vi "0-Draw No-Sail Zones.vi"(4 "Font Size":i16, 5 "Image Descriptor":T2={"Upper-Left Corner Coordinates"={"UTM Zone"=0.0, "Hemisphere"=enum."North", "East"=0.0, "North"=0.0}, "Meters/Pixel"=42.294203} {"Upper-Left Corner Coordinates"."North" format="%#_10f"; "Upper-Left Corner Coordinates"."East" format="%#_8f"}, 6 "No Sail Zone Color":u32(colorbox)=16754450, 7 "No Sail Circles":T1[](array[typedef]), 8 "Image In":T4) -> (1 "Coordinate Outside Image":bool, 3 "Image Out":T4)   [LabVIEW 2011]
doc: "Overlays no-sail zones onto the map image."
uses:
  2-Think/2 Typedefs/UTM Location.ctl
  2-Think/2 Globals/2 Global.vi
  2-Think/2 Classes/Waypoint/Waypoint.lvclass
  <vilib>/vision/Image Controls.llb/IMAQ Image.ctl
  0-Image Descriptor.ctl
  2-Think/2 Typedefs/UTM Circle.ctl
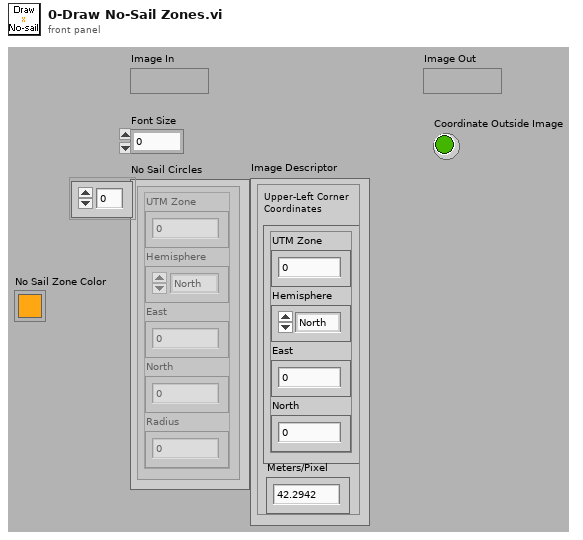
[diagram p1: front panel]
types:
  T1 = typedef "UTM Circle.ctl" = cluster{"UTM Zone":dbl, "Hemisphere":enum16{"North", "South"}, "East":dbl, "North":dbl, "Radius":dbl}
  T2 = typedef "0-Image Descriptor.ctl" = cluster{"Upper-Left Corner Coordinates":T3, "Meters/Pixel":dbl}
  T3 = typedef "UTM Location.ctl" = cluster{"UTM Zone":dbl, "Hemisphere":enum16{"North", "South"}, "East":dbl, "North":dbl}
  T4 = typedef "IMAQ Image.ctl" = refnum<image>
  T5 = cluster{"Desired Font (Application)":enum16{"User-specified Font", "Application Font", "System Font", "Dialog Font"}, "[User-specified Font]":cluster{"Font Name":string, "Size":i16, "Strikeout?":bool, "Italic?":bool, "Underline?":bool, "Outline?":bool, "Shadow?":bool, "Bold?":bool, "Rotation Angle":dbl}, "Horizontal Alignment":i16, "Vertical Alignment":i16}
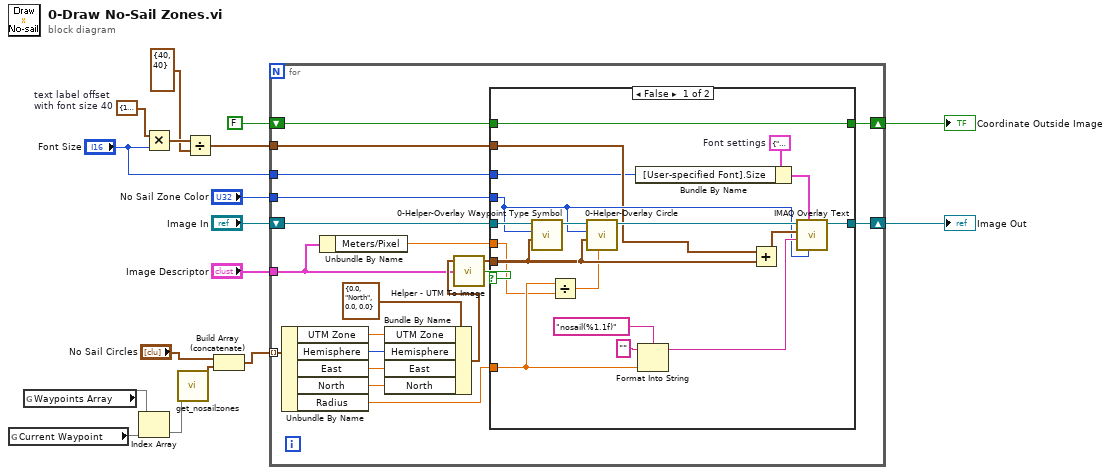
[diagram p0: block diagram]
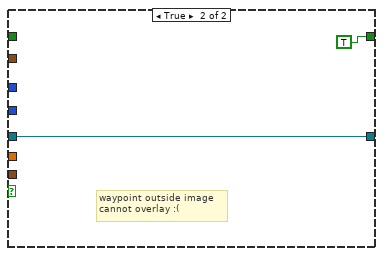
[diagram p2: hidden frame]
diagram:
  w11 = cluster{"X":i32, "Y":i32} {"X"=10, "Y"=21}  # text label offset with font size 40
  n1 = global read "2 Global.vi" "Current Waypoint"() -> (w1)
  n2 = global read "2 Global.vi" "Waypoints Array"() -> (w2)
  n3 = Index Array(array=w2, index=w1) -> (element=w3)
  n4 = Multiply(x=w11, y="Font Size") -> (x*y=w10:cluster{"X":i32, "Y":i32})
  n5 = call-dynamic "get_nosailzones.vi"("Waypoint in"=w3) -> ("No Sail Circles"=w4:T1[])  [unwired: 7 in, 2 out]
  n6 = Divide(x=w10, y=cluster{"X":i32, "Y":i32} {"X"=40, "Y"=40}) -> (x/y=w8:cluster{"X":dbl, "Y":dbl})
  n7 = Build Array (concatenate)("No Sail Circles", w4) -> (w6:T1[])
  n8 = for {
    tunnel: w6 -> [w30] mode=indexing
    shift-right: [w35] -> w16
    shift-left: "Image In" -> [w36]
    tunnel: "Image Descriptor" -> [w21]
    shift-right: [w32] -> w14
    shift-left: FALSE -> [w31]
    tunnel: "No Sail Zone Color" -> [w22]
    tunnel: w8 -> [w19]
    tunnel: "Font Size" -> [w18]
    n9 = Unbundle By Name(w30) -> ("UTM Zone"=w24:dbl, "Hemisphere"=w25:enum16{"North", "South"}, "East"=w26:dbl, "North"=w27:dbl, "Radius"=w29:dbl)
    n10 = Unbundle By Name(w21) -> ("Meters/Pixel"=w20:dbl)
    n11 = Bundle By Name(cluster=T3 {"UTM Zone"=0.0, "Hemisphere"=enum."North", "East"=0.0, "North"=0.0} ("UTM Location"), "UTM Zone"=w24, "Hemisphere"=w25, "East"=w26, "North"=w27) -> (w23:T3)
    n12 = call "Helper - UTM To Image.vi"("Image Descriptor"=w21, "UTM Location"=w23) -> ("Coordinate Outside Image"=w33:bool, "Pixel Coordinates"=w34:cluster{"X":i32, "Y":i32})  [unwired: 1 in, 1 out]
    n13 = case shown="False" w33 {
      tunnel: w36 -> [w49 w56]
      tunnel: [w53 w56] -> w35
      tunnel: w34 -> [w47 _]
      tunnel: [w50 TRUE] -> w32
      tunnel: w31 -> [w50 _]
      tunnel: w29 -> [w42 _]
      tunnel: w22 -> [w44 _]
      tunnel: w20 -> [w41 _]
      tunnel: w19 -> [w38 _]
      tunnel: w18 -> [w37 _]
      frame False {
        w40 = T5 {"Desired Font (Application)"=enum."User-specified Font", "[User-specified Font]"={"Font Name"="Arial Unicode MS", "Size"=40, "Strikeout?"=FALSE, "Italic?"=FALSE, "Underline?"=FALSE, "Outline?"=FALSE, "Shadow?"=FALSE, "Bold?"=TRUE, "Rotation Angle"=0.0}, "Horizontal Alignment"=0, "Vertical Alignment"=0}  # Font settings
        n14 = call "0-Helper-Overlay Waypoint Type Symbol.vi"("Overlay Location"=w47, "Icon Color"=w44, "Image in"=w49) -> ("Image out"=w46:T4)  [unwired: 7 in, 1 out]
        n15 = Divide(x=w42, y=w41) -> (x/y=w43:dbl)
        n16 = call "0-Helper-Overlay Circle.vi"("Radius (px)"=w43, "Pixel Coordinates"=w47, "Color"=w44, "Image in"=w46) -> ("Image out"=w45:T4)  [unwired: 7 in]
        n17 = Bundle By Name(cluster=w40, "[User-specified Font].Size"=w37) -> (w39:T5)
        n18 = Format Into String(format string="nosail(%1.1f)", initial string="", w42) -> (resulting string=w51:string)  [unwired: 1 in, 1 out]
        n19 = Add(x=w38, y=w47) -> (x+y=w54:cluster{"X":dbl, "Y":dbl})
        n20 = call "IMAQ Overlay Text"("Text Color (black)"=w44, "Font, Size & Style"=w39, "String"=w51, "Origin"=w54, "Image"=w45) -> ("Image Out"=w53:T4)  [unwired: 3 in, 3 out]
      }
      frame True {
        # "waypoint outside image\ncannot overlay :("
      }
    }
  }
  "Image Out" <- w16
  "Coordinate Outside Image" <- w14
